vi "New Test (Caraya).vi"   [LabVIEW 2013, in "Caraya.lvlib"]
doc: "Use this method as a template to create a new test case with an assertion.\nThis method is added to the palette and configured to \"Drop VI Content\"."
uses:
  Caraya.lvlib
  Assert True.vi
  Test/Test.lvclass
  Assert.lvclass
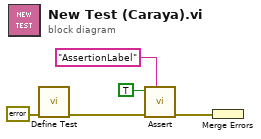
[diagram p0: block diagram]
diagram:
  n1 = call "Define Test.vi"("error in (no error)"=errorcluster {"status"=FALSE, "code"=0, "source"=""}) -> ("error out"=w4:errorcluster)  [unwired: 10 in]
  n2 = call-poly "Assert.vi"("Label"="AssertionLabel" ("Label (VI Title)"), "error in (no error)"=w4, "True?"=TRUE) -> ("error out"=w3:errorcluster)  [unwired: 8 in]
  n3 = Merge Errors(w3) -> ()  [unwired: 1 out]
